vi "updateVariables.vi"(8 "error in (no error)":errorcluster, 11 "AlarmsTreeDisplayTC in":refnum<class "AlarmsTreeDisplayTC.lvclass">) -> (0 "error out":errorcluster, 3 "AlarmsTreeDisplayTC out":refnum<class "AlarmsTreeDisplayTC.lvclass">)   [LabVIEW 2012, in "AlarmsTreeDisplayTC.lvclass"]
doc: "Calls the init method to retrieve the latest shared variable list and initiates listening on those variables."
uses:
  AlarmsTreeDisplayTC.lvclass
  C/Program Files (x86)/National Instruments/LabVIEW 2012/user.lib/Common/AlarmsTreeDisplay/AlarmsTreeDisplay/AlarmsTreeDisplay.lvclass
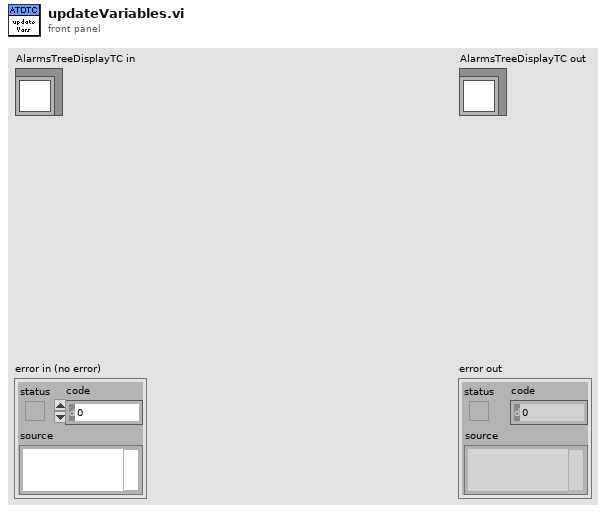
[diagram p1: front panel]
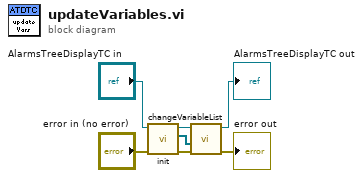
[diagram p0: block diagram]
diagram:
  n1 = call "init.vi"("error in (no error)"="error in (no error)", "AlarmsTreeDisplayTC in"="AlarmsTreeDisplayTC in") -> ("error out"=w3:errorcluster, "shared variables"=w4:refnum<k21>[], "AlarmsTreeDisplayTC out"=w5:refnum<class "AlarmsTreeDisplayTC.lvclass">)  [unwired: 7 in]
  n2 = call "changeVariableList.vi"("error in (no error)"=w3, "shared variables"=w4, "AlarmsTreeDisplay in"=w5) -> ("error out"=→"error out":errorcluster, "AlarmsTreeDisplay out"=→"AlarmsTreeDisplayTC out":refnum<class "AlarmsTreeDisplayTC.lvclass">)  [unwired: 7 in]
